vi "pmu_Check Timestamps Range.vi"(0 "timestamps in":dbl[][](array[numeric]), 11 "GPS information":T1[](array[typedef])) -> (3 "empty?":bool, 4 "timestamps out":dbl[][](array[numeric]), 6 "max initial timestamp":timestamp, 8 "min final timestamp":timestamp, 10 "max t0 index":i32, 15 "buffered GPS information":T1[](array[typedef]))   [LabVIEW 2011, in "NI_EP_PMU.lvlib"]
doc: "This VI updates circular buffer which holds data used later for frequency and phasor calculation. Upon init the buffer size is determined by the size of the incoming waveforms. In subsequent calls the buffer size is kept constant, provided that the size of the incoming waveforms corresponds to elements to read produced by previous iteration of this VI."
uses:
  <vilib>/addons/Electrical Power/PMU/NI_EP_PMU.lvlib
  <vilib>/addons/Electrical Power/PMU/Common/Controls/pmu_GPS Info.ctl
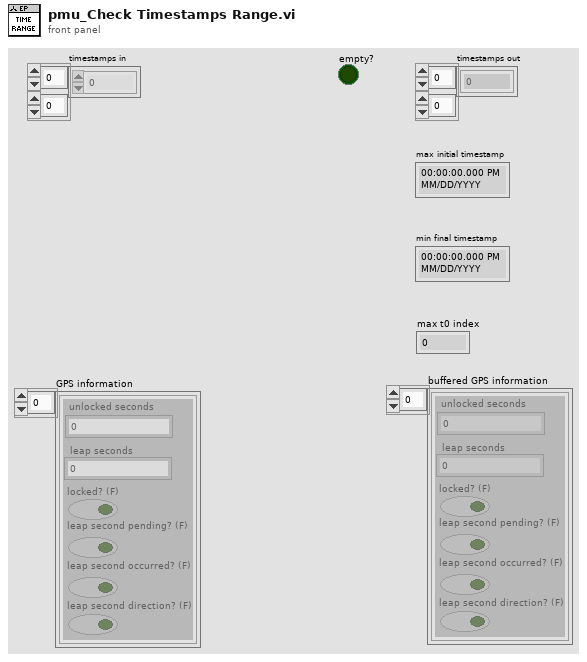
[diagram p1: front panel]
types:
  T1 = typedef "NI_EP_PMU.lvlib/pmu_GPS Info.ctl" = cluster{"unlocked seconds":u32, "leap seconds":i8, "locked? (F)":bool, "leap second pending? (F)":bool, "leap second occurred? (F)":bool, "leap second direction? (F)":bool}
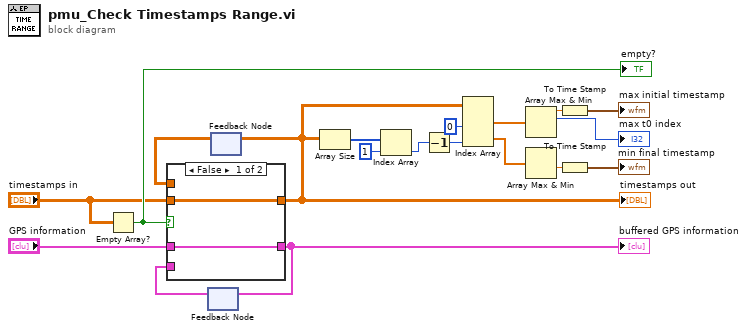
[diagram p0: block diagram]
diagram:
  n1 = Empty Array?(array="timestamps in") -> (empty?=w7:bool)
  "empty?" <- w7
  n2 = feedback #1() -> (w2:T1[])  [unwired: 1 in]
  n3 = feedback #2() -> (w1:dbl[][])  [unwired: 1 in]
  n4 = case shown="False" w7 {
    tunnel: [w21 w22] -> w17
    tunnel: "timestamps in" -> [w21 _]
    tunnel: [w20 w23] -> w3
    tunnel: "GPS information" -> [w20 _]
    tunnel: w2 -> [_ w23]
    tunnel: w1 -> [_ w22]
    frame False {
    }
    frame True {
      # "Empty Array: use the last array"
    }
  }
  "timestamps out" <- w17
  "buffered GPS information" <- w3
  n5 = feedback-in #1(w3) -> ()
  n6 = feedback-in #2(w17) -> ()
  n7 = Array Size(array=w17) -> (size(s)=w10:i32[])
  n8 = Index Array(array=w10, index=1) -> (element=w8:i32)
  n9 = Decrement(x=w8) -> (x-1=w16:i32)
  n10 = Index Array(array=w17, index (col) #1=0 ("disabled index (col)"), index (col) #2=w16) -> (element #1=w14:dbl[], element #2=w12:dbl[])  [unwired: 2 in]
  n11 = Array Max & Min(array=w14) -> (max value=w13:dbl, max index (indices)=→"max t0 index":i32)  [unwired: 2 out]
  n12 = Array Max & Min(array=w12) -> (min value=w11:dbl)  [unwired: 3 out]
  n13 = To Time Stamp(1:w13) -> (0:→"max initial timestamp":timestamp)
  n14 = To Time Stamp(1:w11) -> (0:→"min final timestamp":timestamp)
